vi "Get Channel Variables.vi"(8 "error in (no error)":errorcluster, 9 "Channel":i32, 11 "LabVIEW Web Service Request":refnum<class "Web Request.lvclass">) -> (0 "error out":errorcluster, 3 "LabVIEW Web Service Request out":refnum<class "Web Request.lvclass">)   [LabVIEW 2018]
doc: "This VI sets all of the ESP variables for a single contact so it can be output from an ESP script."
uses:
  <vilib>/wsapi/Web Request.lvclass
  CAEN globals.vi
  subvis/i32 to dec string small.vi
  subvis/bool to string small.vi
  subvis/dbl to fr string small.vi
  <vilib>/wsapi/class/subVIs/Set Many String ESP Variables.vi
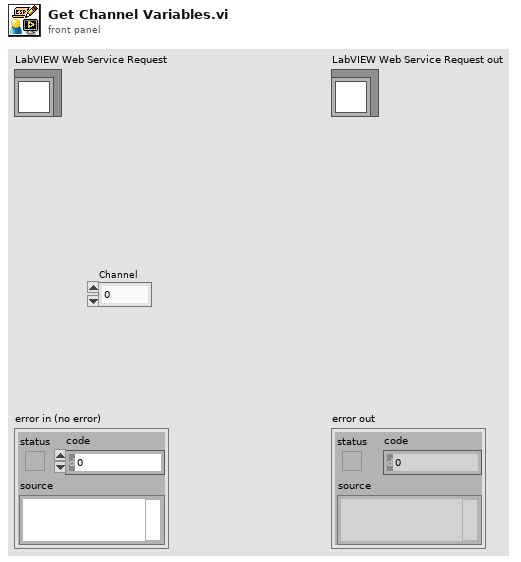
[diagram p1: front panel]
types:
  T1 = typedef "channel_cluster.ctl" = cluster{"Channel Name":string, "Crate":i32, "Card Type":string, "Card":i32, "Channel":i32, "Status Icon":picture, "Vmon (V)":dbl, "Vset (V)":dbl, "Imon (A)":dbl, "Iset (A)":dbl, "Timestamp":string, "ON/OFF":bool, "Status":string, "Vswmax (V)":dbl, "Flag":bool, "Vfile (V)":dbl, "Error Logged":bool[], "enable_file":bool}
  T2 = typedef "crate.ctl" = cluster{"CAENet Address":i32, "Crate Model":string, "Firmware Version":string, "Crate Map":T3[], "Total Channels":i32}
  T3 = typedef "card.ctl" = cluster{"Slot Number":i32, "Card Model":string, "Num Channels":i32, "Polarity":string, "Vmax":dbl, "Imax":dbl, "Revision":string}
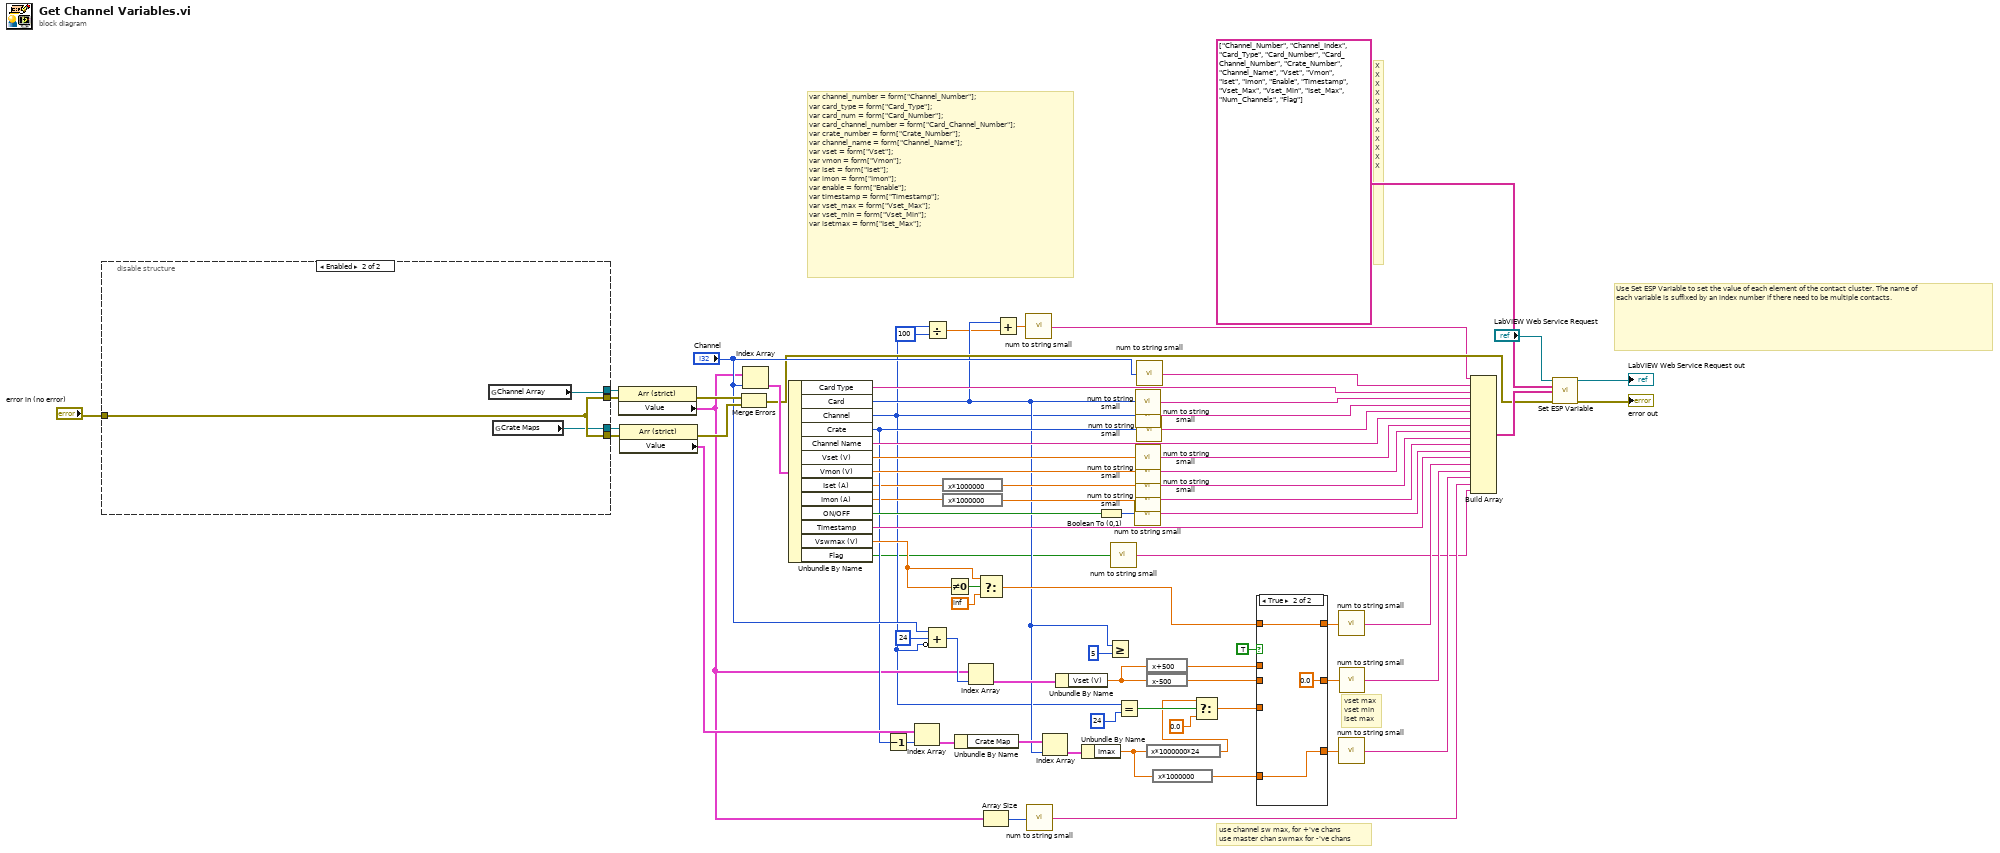
[diagram p0: block diagram]
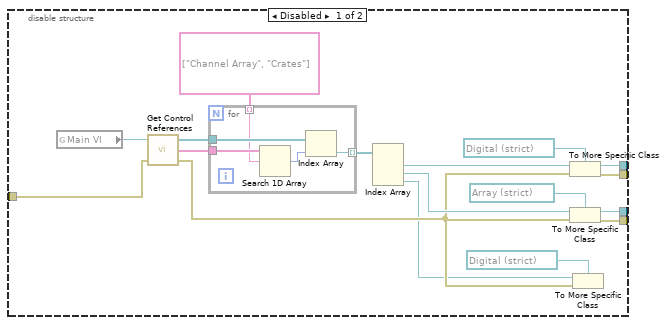
[diagram p3: hidden frame]
diagram:
  # "vset max\nvset min\niset max"
  # "X\nX\nX\nX\nX\nX\nX\nX\nX\nX\nX\nX"
  # "use channel sw max, for +'ve chans\nuse master chan swmax for -'ve chans"
  # "var channel_number = form[\"Channel_Number\"];\nvar card_type = form[\"Card_Type\"];\nvar card_num = form[\"Card_Number\"];\nvar card_channel_number = form[\"Card_Channel_Number\"];\nvar crate_number = form[\"Crate_Number\"];\nvar channel_name = form[\"Channel_Name\"];\nvar vset = form[\"Vset\"];\nvar vmon = form[\"Vmon\"];\nvar iset = form[\"Iset\"];\nvar imon = form[\"Imon\"];\nvar enable = form[\"Enable\"];\nvar timestamp = form[\"Timestamp\"];\nvar vset_max = form[\"Vset_Max\"];\nvar vset_min = form[\"Vset_Min\"];\nvar isetmax = form[\"Iset_Max\"];"
  # "Use Set ESP Variable to set the value of each element of the contact cluster. The name of each variable is suffixed by an index number if there need to be multiple contacts."
  n1 = disable-structure shown="Enabled" {
    disable-tunnel: [w86 w100] -> w77
    disable-tunnel: [w85 w102] -> w76
    disable-tunnel: [w83 w101] -> w75
    disable-tunnel: [w82 w102] -> w74
    disable-tunnel: "error in (no error)" -> [w78 w102]
    frame Disabled {
      n2 = global read "CAEN globals.vi" "Main VI"() -> (w94:refnum<vi>)
      n3 = call "Get Control References.vi"("error in"=w78, "This vi"=w94) -> ("error out"=w80:errorcluster, "Control Names"=w93:string[], "Controls[]"=w92:refnum<vi>[])  [unwired: 1 in]
      n4 = for {
        tunnel: w93 -> [w99]
        tunnel: w92 -> [w97]
        tunnel: [w96] -> w90 mode=indexing
        tunnel: string[] ["Channel Array", "Crates"] ("Control Names") -> [w95] mode=indexing
        n5 = Search 1D Array(1D array=w99, element=w95) -> (index of element=w98:i32)  [unwired: 1 in]
        n6 = Index Array(array=w97, index=w98) -> (element=w96:refnum<vi>)
      }
      n7 = Index Array(array=w90) -> (element #1=w88:refnum<vi>, element #2=w84:refnum<vi>, element #3=w79:refnum<vi>)  [unwired: 3 in]
      n8 = To More Specific Class(target class=refnum<vi> refnum ("History Length"), reference=w88, error in=w80) -> (specific class reference=w83:refnum<vi>, error out=w82:errorcluster)
      n9 = To More Specific Class(target class=refnum<vi> refnum ("Channel Array"), reference=w84, error in=w80) -> (specific class reference=w86:refnum<vi>, error out=w85:errorcluster)
      n10 = To More Specific Class(target class=refnum<vi> refnum ("History Length"), reference=w79, error in=w80) -> ()  [unwired: 2 out]
    }
    frame Enabled {
      n11 = global read "CAEN globals.vi" "Channel Array"() -> (w101:refnum<vi>)
      n12 = global read "CAEN globals.vi" "Crate Maps"() -> (w100:refnum<vi>)
    }
  }
  n13 = property class="Arr (strict)"(reference=w75, error in=w74) -> (error out=w73:errorcluster, "Value"=w26:T1[])  [unwired: 1 out]
  n14 = property class="Arr (strict)"(reference=w77, error in=w76) -> (error out=w72:errorcluster, "Value"=w44:T2[])  [unwired: 1 out]
  n15 = Merge Errors(w73, w72) -> (w18:errorcluster)
  n16 = Index Array(array=w26, index="Channel") -> (element=w64:T1)
  n17 = Unbundle By Name(w64) -> ("Card Type"=w50:string, "Card"=w17:i32, "Channel"=w12:i32, "Crate"=w28:i32, "Channel Name"=w60:string, "Vset (V)"=w59:dbl, "Vmon (V)"=w40:dbl, "Iset (A)"=w22:dbl, "Imon (A)"=w20:dbl, "ON/OFF"=w35:bool, "Timestamp"=w32:string, "Vswmax (V)"=w56:dbl, "Flag"=w3:bool)
  n18 = Decrement(x=w28) -> (x-1=w27:i32)
  n19 = Index Array(array=w44, index=w27) -> (element=w43:T2)
  n20 = Divide(x=w12, y=100) -> (x/y=w13:dbl)
  n21 = Compound Arithmetic op=ADD("Channel", 24 ("value"), invert w12) -> (w52:i32)
  n22 = expression code="x*1000000"(w22) -> (w21:dbl)
  n23 = expression code="x*1000000"(w20) -> (w19:dbl)
  n24 = Not Equal To 0?(x=w56) -> (x != 0?=w57:bool)
  n25 = Unbundle By Name(w43) -> ("Crate Map"=w42:T3[])
  n26 = Index Array(array=w26, index=w52) -> (element=w51:T1)
  n27 = Select(t=w56, s=w57, f=inf) -> (s? t:f=w47:dbl)
  n28 = Array Size(array=w26) -> (size(s)=w25:i32)
  n29 = Add(x=w17, y=w13) -> (x+y=w16:dbl)
  n30 = call-poly "num to string small.vi"("number"=w16) -> ("String"=w15:string)  [unwired: 14 in]
  n31 = call-poly "num to string small.vi"("number"=w25) -> ("String"=w24:string)  [unwired: 14 in]
  n32 = Index Array(array=w42, index=w17) -> (element=w41:T3)
  n33 = Unbundle By Name(w51) -> ("Vset (V)"=w49:dbl)
  n34 = Unbundle By Name(w41) -> ("Imax"=w5:dbl)
  n35 = Boolean To (0,1)(Boolean=w35) -> (0, 1=w34:i16)
  n36 = Greater Or Equal?(x=w17, y=5) -> ()  [unwired: 1 out]
  n37 = call-poly "num to string small.vi"("number"=w3) -> ("String"=w2:string)  [unwired: 14 in]
  n38 = Equal?(x=w12, y=24) -> (x = y?=w9:bool)
  n39 = call-poly "num to string small.vi"("number"=w34) -> ("String"=w33:string)  [unwired: 14 in]
  n40 = call-poly "num to string small.vi"("number"=w17) -> ("String"=w63:string)  [unwired: 14 in]
  n41 = call-poly "num to string small.vi"("number"=w12) -> ("String"=w62:string)  [unwired: 14 in]
  n42 = call-poly "num to string small.vi"("number"=w59) -> ("String"=w58:string)  [unwired: 14 in]
  n43 = call-poly "num to string small.vi"("number"=w40) -> ("String"=w39:string)  [unwired: 14 in]
  n44 = call-poly "num to string small.vi"("number"=w21) -> ("String"=w38:string)  [unwired: 14 in]
  n45 = call-poly "num to string small.vi"("number"=w19) -> ("String"=w36:string)  [unwired: 14 in]
  n46 = call-poly "num to string small.vi"("number"=w28) -> ("String"=w61:string)  [unwired: 14 in]
  n47 = call-poly "num to string small.vi"("number"="Channel") -> ("String"=w71:string)  [unwired: 14 in]
  n48 = expression code="x*1000000*24"(w5) -> (w6:dbl)
  n49 = expression code="x+500"(w49) -> (w48:dbl)
  n50 = expression code="x-500"(w49) -> (w10:dbl)
  n51 = expression code="x*1000000"(w5) -> (w4:dbl)
  n52 = Select(t=w6, s=w9, f=0.0) -> (s? t:f=w8:dbl)
  n53 = case shown="True" TRUE {
    tunnel: w48 -> [w105 _]
    tunnel: w10 -> [w104 _]
    tunnel: w47 -> [_ w108]
    tunnel: [w105 w108] -> w46
    tunnel: [w104 0.0 ("Vset (V)")] -> w45
    tunnel: w8 -> [w103 _]
    tunnel: [w103 w106] -> w37
    tunnel: w4 -> [_ w106]
    frame False {
    }
    frame True {
    }
  }
  n54 = call-poly "num to string small.vi"("number"=w46) -> ("String"=w31:string)  [unwired: 14 in]
  n55 = call-poly "num to string small.vi"("number"=w37) -> ("String"=w29:string)  [unwired: 14 in]
  n56 = call-poly "num to string small.vi"("number"=w45) -> ("String"=w30:string)  [unwired: 14 in]
  n57 = Build Array(w15, w71, w50, w63, w62, w61, w60, w58, w39, w38, w36, w33, w32, w31, w30, w29, w24, w2) -> (w69:string[])
  n58 = call-poly <vilib>:"Set ESP Variable.vi"("LabVIEW Web Service Request"="LabVIEW Web Service Request", "keys"=string[] ["Channel_Number", "Channel_Index", "Card_Type", "Card_Number", "Card_Channel_Number", "Crate_Number", "Channel_Name", "Vset", "Vmon", "Iset", "Imon", "Enable", "Timestamp", "Vset_Max", "Vset_Min", "Iset_Max", "Num_Channels", "Flag"] ("appended array"), "values"=w69, "error in (no error)"=w18) -> ("LabVIEW Web Service Request out"=→"LabVIEW Web Service Request out":refnum<class "Web Request.lvclass">, "error out"=→"error out":errorcluster)  [unwired: 10 in]
